vi "Ridimensiona tabella.vi"(11 "Array":string[][](array[string])) -> (3 "Array 2":string[][](array[string]))   [LabVIEW 2016]
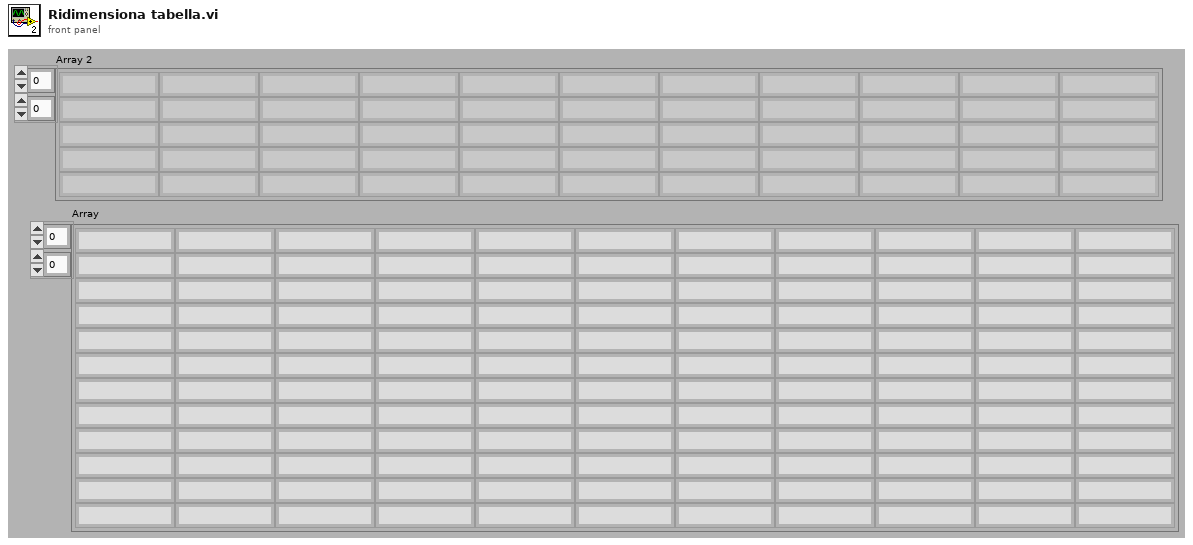
[diagram p1: front panel]
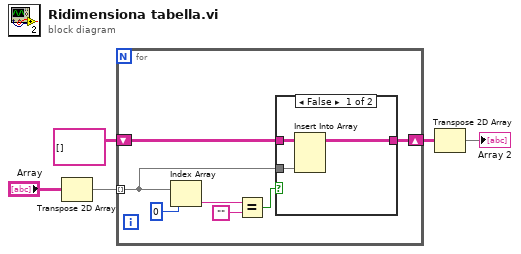
[diagram p0: block diagram]
diagram:
  n1 = Transpose 2D Array(2D array="Array") -> (transposed array=w1:string[][])
  n2 = for {
    tunnel: w1 -> [w7] mode=indexing
    shift-right: [w8] -> w5
    shift-left: string[][] [] -> [w9]
    n3 = Index Array(array=w7, index=0) -> (element=w11:string)
    n4 = Equal?(x=w11, y="") -> (x = y?=w10:bool)
    n5 = case shown="False" w10 {
      tunnel: w9 -> [w15 w16]
      tunnel: [w14 w16] -> w8
      tunnel: w7 -> [w13 _]
      frame False {
        n6 = Insert Into Array "Insert Into Array"(array=w15, new element=w13) -> (w14:string[][])  [unwired: 2 in]
      }
      frame True {
      }
    }
  }
  n7 = Transpose 2D Array(2D array=w5) -> (transposed array=→"Array 2":string[][])
